vi "Untitled 6.vi"() -> ()   [LabVIEW 2017]
uses:
  <vilib>/myRIO/Instrument Drivers/Onboard IO/PWM/typedefs/PWM Reference.ctl
  <vilib>/myRIO/Common/Instrument Driver Framework/Utilities/typedefs/myRIO Generic Hardware Reference.ctl
  <vilib>/myRIO/Common/Instrument Driver Framework/Utilities/typedefs/Hardware Version Enum.ctl
  <vilib>/myRIO/Common/Instrument Driver Framework/Utilities/typedefs/myRIO v1.0 Reference.ctl
  <vilib>/myRIO/Common/Instrument Driver Framework/Utilities/typedefs/Generic FPGA Reference.ctl
  <vilib>/myRIO/Common/Instrument Driver Framework/myRIO v1.0/PWM/typedefs/PWM Channels Enum.ctl
  <vilib>/myRIO/Instrument Drivers/Onboard IO/PWM/typedefs/PWM Configuration.ctl
  <vilib>/userdefined/High Color/nirio_resource_hc.ctl
  <vilib>/myRIO/Instrument Drivers/Onboard IO/DIO/typedefs/DIO Reference.ctl
  <vilib>/myRIO/Common/Instrument Driver Framework/myRIO v1.0/DIO/typedefs/DIO Channels List.ctl
  <vilib>/myRIO/Common/Instrument Driver Framework/myRIO v1.0/DIO/typedefs/DIO Channels Enum.ctl
  <vilib>/myRIO/Common/Instrument Driver Framework/Utilities/vis/Is FPGA Ref Available.vi
  <vilib>/myRIO/Common/Instrument Driver Framework/myRIO v1.0/PWM/vis/myRIO v1.1 Open PWM.vi
  <vilib>/myRIO/Instrument Drivers/Onboard IO/PWM/vis/Set Duty Cycle and Frequency.vi
  <vilib>/myRIO/Common/Instrument Driver Framework/myRIO v1.0/DIO/vis/myRIO v1.1 Open DIO.vi
  <vilib>/myRIO/Common/Instrument Driver Framework/Utilities/vis/Validate Channels.vi
  <vilib>/myRIO/Common/Instrument Driver Framework/myRIO v1.0/PWM/vis/myRIO v1.0 Reserve PWM.vi
  <vilib>/myRIO/Common/Instrument Driver Framework/myRIO v1.0/DIO/vis/myRIO v1.0 Reserve DIO.vi
  <vilib>/myRIO/Common/Instrument Driver Framework/myRIO v1.0/DIO/vis/myRIO v1.0 Close DIO.vi
  <vilib>/myRIO/Common/Instrument Driver Framework/myRIO v1.0/UART/vis/myRIO v1.0 Close UART.vi
  <vilib>/myRIO/Common/Instrument Driver Framework/myRIO v1.0/PWM/vis/myRIO v1.0 Build MUX Configuration PWM.vi
  <vilib>/myRIO/Common/Instrument Driver Framework/myRIO v1.0/Resource Manager/vis/myRIO v1.0 Reserve Channel List.vi
  <vilib>/myRIO/Common/Instrument Driver Framework/myRIO v1.0/DIO/vis/myRIO v1.0 Build MUX Configuration DIO.vi
  <vilib>/myRIO/Common/Instrument Driver Framework/myRIO v1.0/DIO/vis/myRIO v1.0 Unreserve DIO.vi
  <vilib>/myRIO/Common/Instrument Driver Framework/myRIO v1.0/Resource Manager/vis/myRIO v1.0 Create Configuration List.vi
  <vilib>/myRIO/Common/Instrument Driver Framework/myRIO v1.0/Resource Manager/vis/myRIO v1.0 Reserve Channel.vi
  <vilib>/myRIO/Common/Instrument Driver Framework/myRIO v1.0/Resource Manager/vis/myRIO v1.0 Unreserve Channel.vi
  <vilib>/myRIO/Common/Instrument Driver Framework/myRIO v1.0/Resource Manager/vis/myRIO v1.0 Unreserve Channel List.vi
  <vilib>/myRIO/Common/Instrument Driver Framework/myRIO v1.0/Resource Manager/vis/myRIO v1.0 Build Mutex Name.vi
  <vilib>/Utility/VariantDataType/GetNumericInfo.vi
  <vilib>/Utility/error.llb/Error Cluster From Error Code.vi
  <vilib>/myRIO/Common/Instrument Driver Framework/myRIO v1.0/myRIO v1.1 Open.vi
  <vilib>/myRIO/Common/Instrument Driver Framework/Utilities/vis/IO Manager.vi
  <vilib>/myRIO/Common/Instrument Driver Framework/Utilities/vis/Configuration Manager.vi
  <vilib>/myRIO/Common/Instrument Driver Framework/myRIO v1.0/Resource Manager/vis/myRIO v1.0 Configure IO.vi
  <vilib>/myRIO/Common/Instrument Driver Framework/myRIO v1.0/myRIO v1.0 Close.vi
  <vilib>/myRIO/Common/Instrument Driver Framework/myRIO v1.0/PWM/vis/myRIO v1.0 Write PWM.vi
  <vilib>/myRIO/Common/Instrument Driver Framework/myRIO v1.0/DIO/vis/myRIO v1.0 Write DIO.vi
  <vilib>/myRIO/Common/Instrument Driver Framework/myRIO v1.0/DIO/vis/myRIO v1.0 Read DIO.vi
  <vilib>/myRIO/Common/Instrument Driver Framework/myRIO v1.0/DIO/vis/myRIO v1.0 Shutdown DIO.vi
  <vilib>/myRIO/Common/Instrument Driver Framework/Utilities/vis/FPGA Ref Manager.vi
  <vilib>/myRIO/Common/Instrument Driver Framework/myRIO v1.0/myRIO v1.0 Reset FPGA.vi
  <vilib>/myRIO/Common/Instrument Driver Framework/myRIO v1.0/IRQ/vis/myRIO v1.0 IRQ Info FGV.vi
  <vilib>/myRIO/Common/Instrument Driver Framework/myRIO v1.0/IRQ/vis/myRIO v1.0 Timer IRQ Info FGV.vi
  <vilib>/myRIO/Common/Instrument Driver Framework/myRIO v1.0/IRQ/vis/myRIO v1.0 ISR Agent.vi
  <vilib>/myRIO/Express VI/Onboard IO/PWM/PWM Express VI.xnode
  <vilib>/myRIO/Instrument Drivers/Onboard IO/PWM/vis/myRIO PWM Open.xnode
  <vilib>/myRIO/Express VI/Onboard IO/DO/DO Express VI.xnode
  <vilib>/myRIO/Instrument Drivers/Onboard IO/DIO/vis/myRIO DIO Open.xnode
  <vilib>/myRIO/Express VI/Onboard Devices/LED/LED Express VI.xnode
  <vilib>/myRIO/Instrument Drivers/Utilities/Utilities.lvlib
  <vilib>/myRIO/Instrument Drivers/Onboard IO/DIO/DIO.lvlib
  <vilib>/myRIO/Instrument Drivers/Onboard IO/PWM/PWM.lvlib
panel:
  in  "Angle":dbl
  in  "Numeric":dbl
  in  "error in (no error)":errorcluster
  in  "myRIO DIO Channel":tag="C/DIO1"
  in  "Temperature (deg C)":dbl=25.0
  out "Distance (cm)":dbl
  in  "stop":bool
  in  "fwd":bool
  out "error out":errorcluster
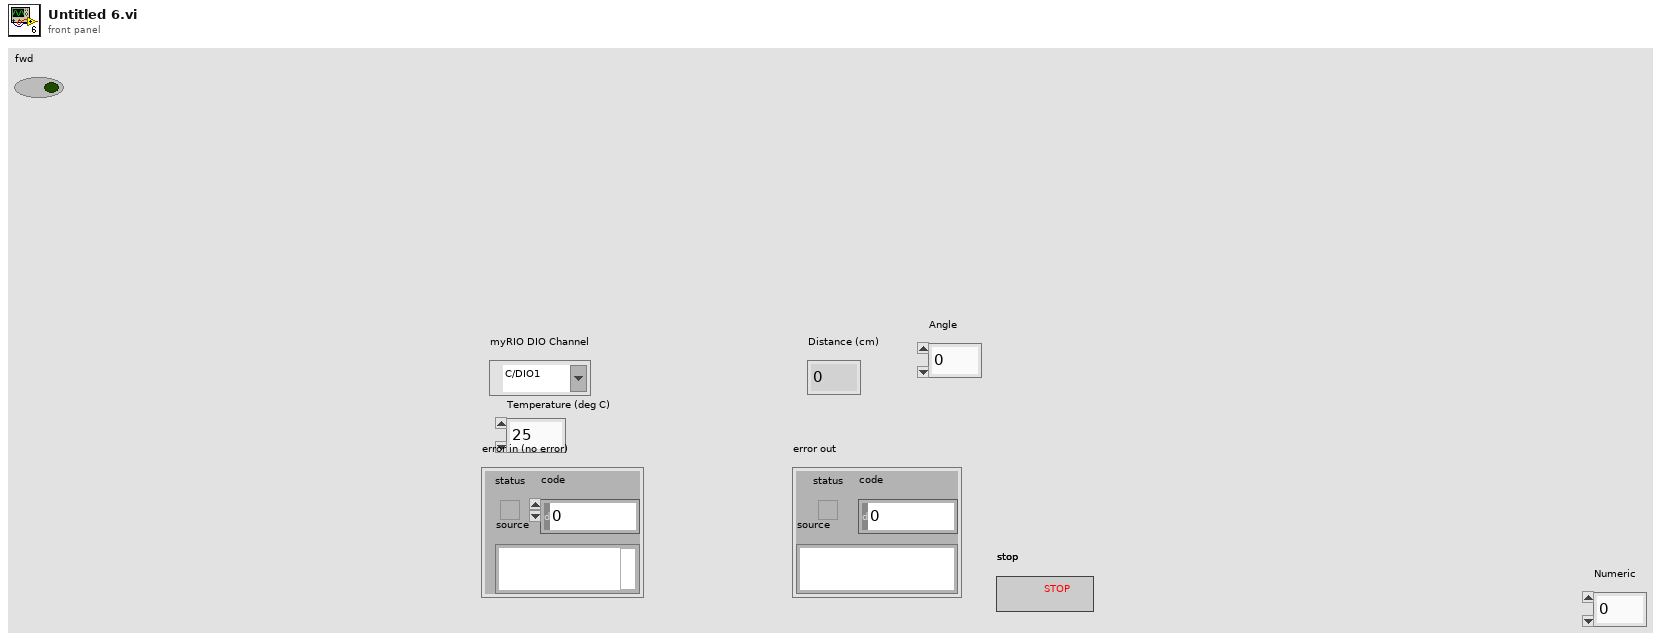
[diagram p1: front panel]
types:
  T1 = enum16{"Initialize", "Trigger pulse", "Wait for rising edge", "Wait for falling edge", "Calculate distance", "Stop"}
  T2 = typedef "DIO.lvlib/DIO Reference.ctl" = cluster{"myRIO Reference":T3, "DIO Channels List":T7}
  T3 = typedef "myRIO Generic Hardware Reference.ctl" = cluster{"myRIO Model":T4, "myRIO Hardware Reference":T5}
  T4 = typedef "Hardware Version Enum.ctl" = enum16{"Unknown", "myRIO-1900", "myRIO-1950", "roboRIO", "NI ELVIS RIO CM"}
  T5 = typedef "myRIO v1.0 Reference.ctl" = cluster{"Generic FPGA Reference":T6, "Allow multiple opens":bool}
  T6 = typedef "Generic FPGA Reference.ctl" = refnum<k20>
  T7 = typedef "DIO Channels List.ctl" = T8[]
  T8 = typedef "DIO Channels Enum.ctl" = enum16{"Not Connected", "C/DIO0", "C/DIO1", "C/DIO2", "C/DIO3", "C/DIO4", "C/DIO5", "C/DIO6", "C/DIO7", "A/DIO0", "A/DIO1", "A/DIO2", "A/DIO3", "A/DIO4", "A/DIO5", "A/DIO6", "A/DIO7", "A/DIO8", "A/DIO9", "A/DIO10", "A/DIO11", "A/DIO12", "A/DIO13", "A/DIO14", "A/DIO15", "B/DIO0", "B/DIO1", "B/DIO2", "B/DIO3", "B/DIO4", "B/DIO5", "B/DIO6", "B/DIO7", "B/DIO8", "B/DIO9", "B/DIO10", "B/DIO11", "B/DIO12", "B/DIO13", "B/DIO14", "B/DIO15", "LED0", "LED1", "LED2", "LED3", "Button0", "DIO/DIO0", "DIO/DIO1", "DIO/DIO2", "DIO/DIO3", "DIO/DIO4", "DIO/DIO5", "DIO/DIO6", "DIO/DIO7", "DIO/DIO8", "DIO/DIO9", "SPI/CS0", "SPI/CS1", "SPI/CS2", "SPI/CS3", "LED RADIO (Green)", "LED RADIO (Red)", "LED COMM (Green)", "LED COMM (Red)", "LED MODE (Green)", "LED MODE (Red)"}
  T9 = typedef "nirio_resource_hc.ctl" = tag
  T10 = typedef "PWM.lvlib/PWM Reference.ctl" = cluster{"myRIO Reference":T3, "PWM Channels Enum":T11, "PWM Configuration":T12}
  T11 = typedef "PWM Channels Enum.ctl" = enum16{"Not Connected", "C/PWM0", "C/PWM1", "A/PWM0", "A/PWM1", "A/PWM2", "B/PWM0", "B/PWM1", "B/PWM2", "PWM/PWM0", "PWM/PWM1", "PWM/PWM2", "PWM/PWM3", "PWM/PWM4", "PWM/PWM5", "PWM/PWM6", "PWM/PWM7", "PWM/PWM8", "PWM/PWM9"}
  T12 = typedef "PWM.lvlib/PWM Configuration.ctl" = cluster{"Frequency":dbl, "Duty Cycle":dbl}
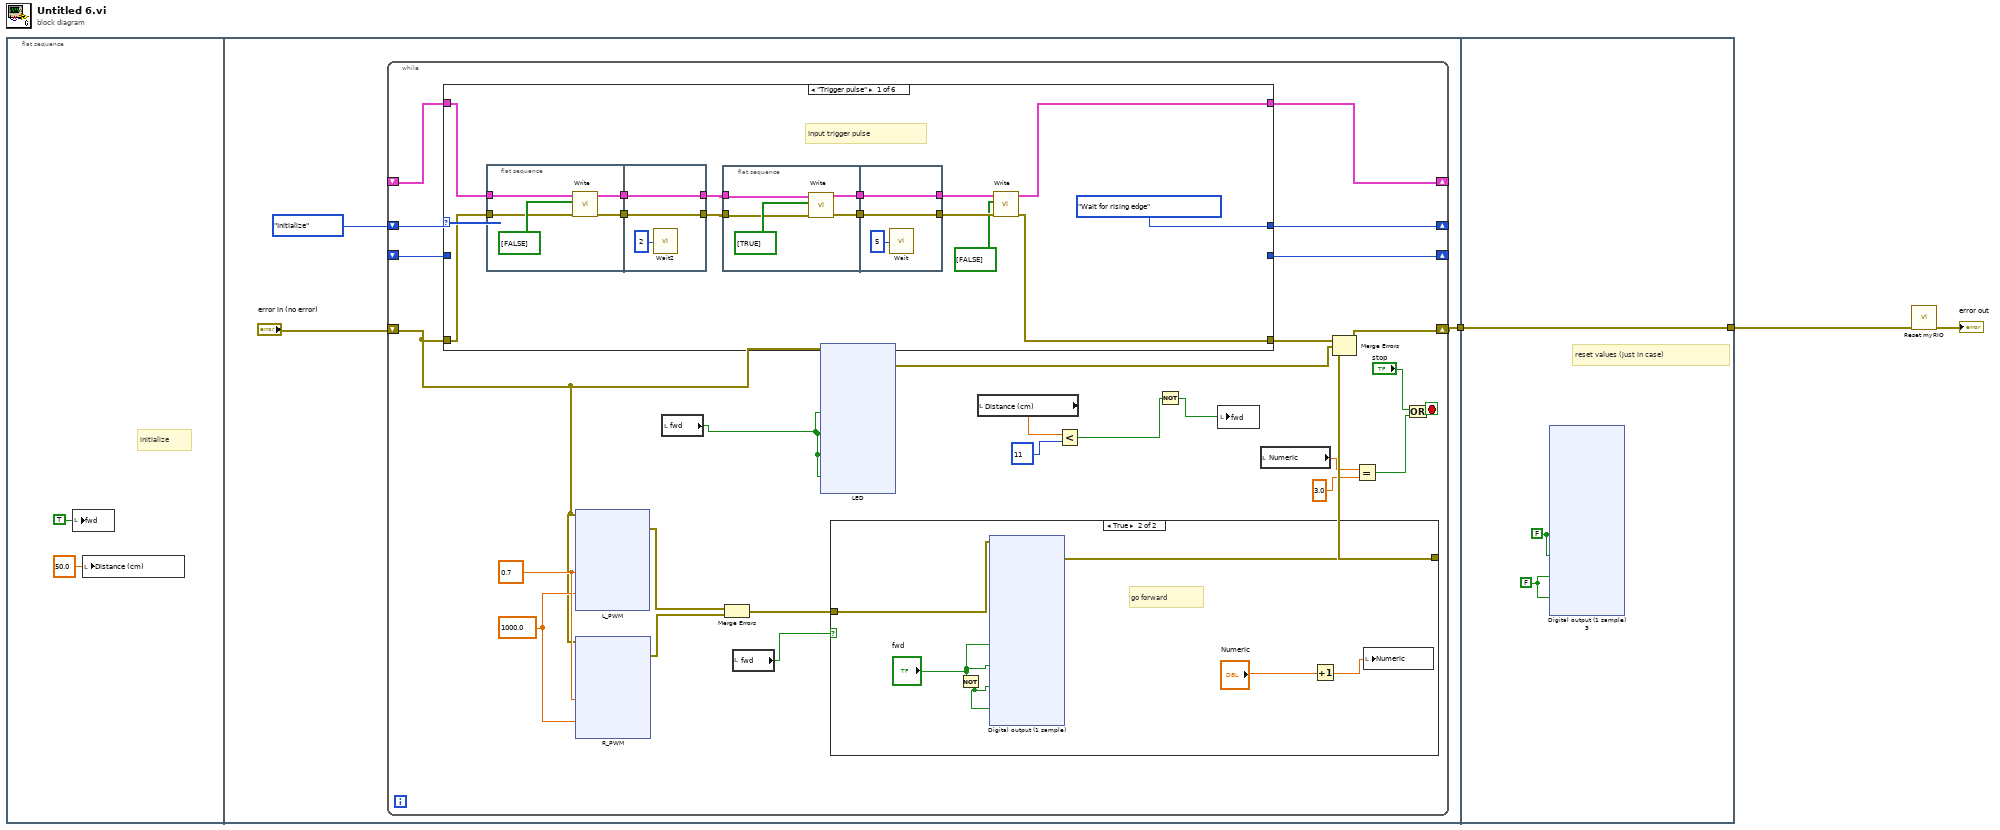
[diagram p0: block diagram]
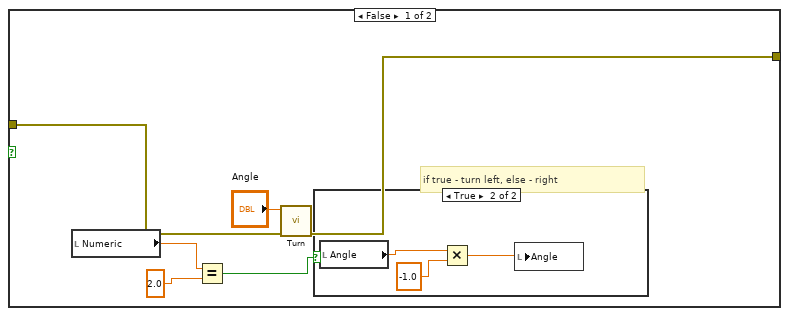
[diagram p2: hidden frame]
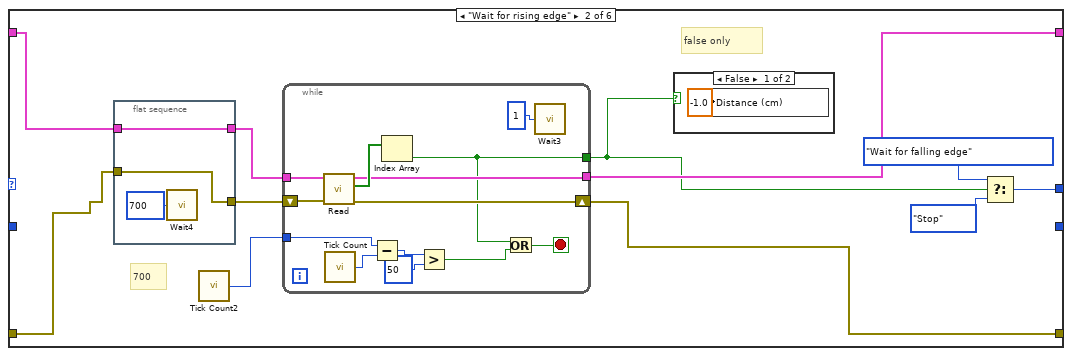
[diagram p4: hidden frame]
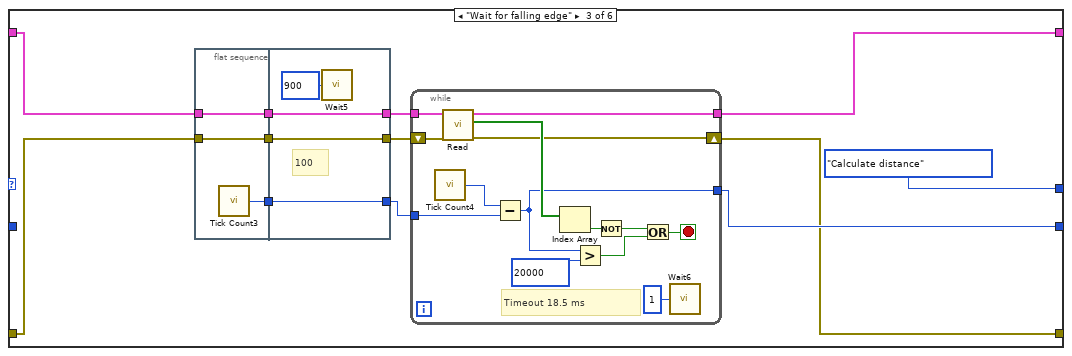
[diagram p6: hidden frame]
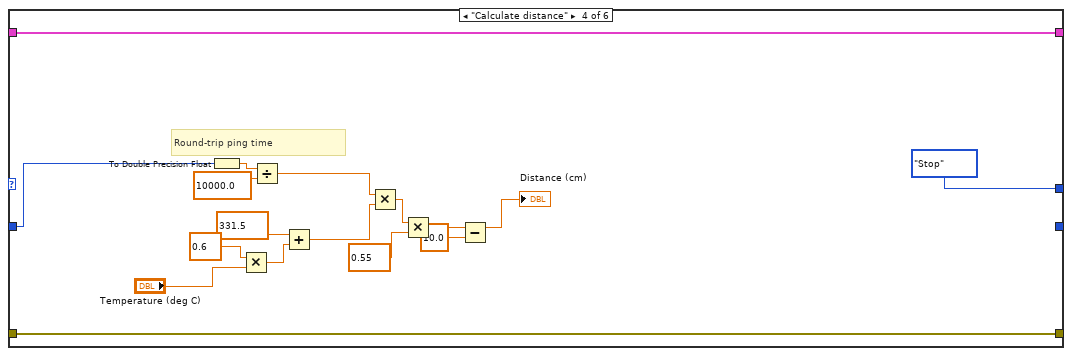
[diagram p7: hidden frame]
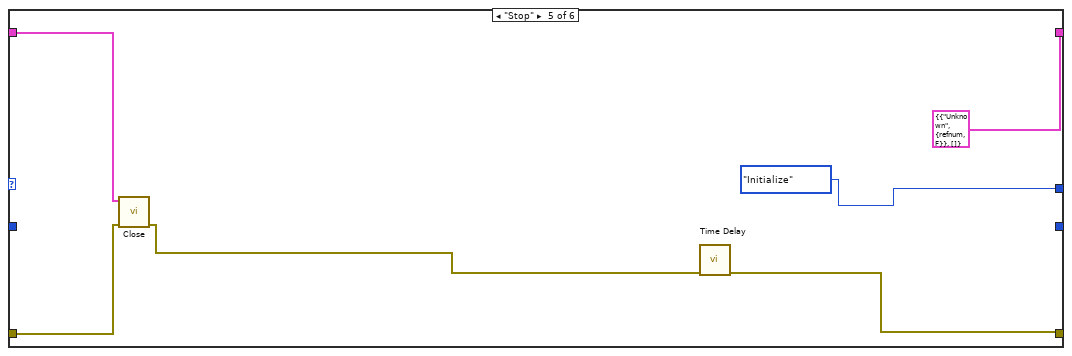
[diagram p8: hidden frame]
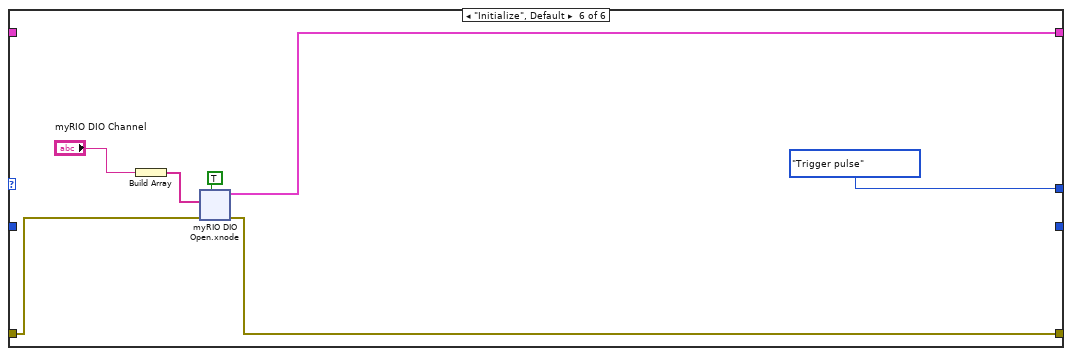
[diagram p9: hidden frame]
diagram:
  n1 = flat-sequence {
    tunnel: [w6] -> w1
    tunnel: [w336] -> w3
    tunnel: w1 -> [w336]
    frame #0 {
      # "initialize"
      n2 = local write "fwd"(TRUE ("fwd")) -> ()
      n3 = local write "Distance (cm)"(50.0 ("Distance (cm)")) -> ()
    }
    frame #1 {
      n4 = while {
        shift-right: [w30] -> _
        shift-left: T1."Initialize" -> [w35]
        shift-right: [w27] -> w6
        shift-left: "error in (no error)" -> [w19]
        shift-right: [w34] -> _
        shift-left: _ -> [w33]
        shift-right: [w29] -> _
        shift-left: _ -> [w31]
        stop <- w18 stop-if-true
        w22 = 1000.0 ("Frequency [Hz]")
        w23 = 0.7 ("Duty Cycle")
        n5 = case shown="\"Trigger pulse\"" w35 {
          tunnel: [T1."Wait for rising edge" w228 T1."Calculate distance" ("y") T1."Stop" ("y") T1."Initialize" ("y") T1."Trigger pulse"] -> w30
          tunnel: w19 -> [w201 w233 w259 w292 w310 w315]
          tunnel: [w199 w237 w258 w304 T2 {"myRIO Reference"={"myRIO Model"=enum."Unknown", "myRIO Hardware Reference"={"Generic FPGA Reference"=refnum, "Allow multiple opens"=FALSE}}, "DIO Channels List"=[]} ("DIO Ref Out") w314] -> w34
          tunnel: w33 -> [w200 w232 w260 w304 w309 _]
          tunnel: [w198 w236 w255 w292 w305 w313] -> w32
          tunnel: [_ _ w257 _ _ _] -> w29
          tunnel: w31 -> [_ _ _ w291 _ _]
          frame "Trigger pulse" {
            # "Input trigger pulse"
            n6 = flat-sequence {
              tunnel: [w214] -> w208
              tunnel: [w213] -> w207
              tunnel: w201 -> [w212]
              tunnel: w200 -> [w211]
              tunnel: [w217] -> w205
              tunnel: [w216] -> w206
              tunnel: w208 -> [w217]
              tunnel: w207 -> [w216]
              frame #0 {
                n7 = call <vilib>:"Write.vi"("error in (no error)"=w212, "Values"=bool[] [FALSE], "DIO Ref In"=w211) -> ("error out"=w213:errorcluster, "DIO Ref Out"=w214:T2)  [unwired: 6 in]
              }
              frame #1 {
                n8 = call "Wait2"("Count(uSec)"=u32 2) -> ()  [unwired: 1 out]
              }
            }
            n9 = flat-sequence {
              tunnel: [w222] -> w210
              tunnel: [w221] -> w209
              tunnel: w206 -> [w220]
              tunnel: w205 -> [w219]
              tunnel: [w225] -> w202
              tunnel: [w224] -> w204
              tunnel: w210 -> [w225]
              tunnel: w209 -> [w224]
              frame #0 {
                n10 = call <vilib>:"Write.vi"("error in (no error)"=w220, "Values"=bool[] [TRUE], "DIO Ref In"=w219) -> ("error out"=w221:errorcluster, "DIO Ref Out"=w222:T2)  [unwired: 6 in]
              }
              frame #1 {
                n11 = call "Wait"("Count(uSec)"=u32 5) -> ()  [unwired: 1 out]
              }
            }
            n12 = call <vilib>:"Write.vi"("error in (no error)"=w204, "Values"=bool[] [FALSE], "DIO Ref In"=w202) -> ("error out"=w198:errorcluster, "DIO Ref Out"=w199:T2)  [unwired: 6 in]
          }
          frame "Wait for rising edge" {
            # "700"
            # "false only"
            n13 = flat-sequence {
              tunnel: [w240] -> w234
              tunnel: w233 -> [w240]
              tunnel: w232 -> [w239]
              tunnel: [w239] -> w231
              frame #0 {
                n14 = call "Wait4"("Count(uSec)"=u32 700) -> ()  [unwired: 1 out]
              }
            }
            n15 = call "Tick Count2"() -> ("Tick Count(uSec)"=w235:u32)
            n16 = while {
              tunnel: [w252] -> w237
              shift-right: [w250] -> w236
              shift-left: w234 -> [w251]
              tunnel: w235 -> [w247]
              tunnel: w231 -> [w249]
              tunnel: [w242] -> w227
              stop <- w244 stop-if-true
              n17 = call <vilib>:"Read.vi"("error in (no error)"=w251, "DIO Ref In"=w249) -> ("error out"=w250:errorcluster, "Values"=w253:bool[], "DIO Ref Out"=w252:T2)  [unwired: 7 in]
              n18 = call "Tick Count"() -> ("Tick Count(uSec)"=w248:u32)
              n19 = Subtract(x=w247, y=w248) -> (x-y=w246:u32)
              n20 = Index Array(array=w253) -> (element=w242:bool)  [unwired: 1 in]
              n21 = Greater?(x=w246, y=u32 50) -> (0:w243:bool)
              n22 = Or(x=w242, y=w243) -> (x .or. y?=w244:bool)
              n23 = call "Wait3"("Count(uSec)"=u32 1) -> ()  [unwired: 1 out]
            }
            n24 = case shown="False" w227 {
              frame False {
                n25 = local write "Distance (cm)"(-1.0 ("Distance (m)")) -> ()
              }
              frame True {
              }
            }
            n26 = Select(t=T1."Wait for falling edge", s=w227, f=T1."Stop" ("y")) -> (s? t:f=w228:T1)
          }
          frame "Wait for falling edge" {
            n27 = flat-sequence {
              tunnel: w260 -> [w283]
              tunnel: [w283] -> w266
              tunnel: [w282] -> w265
              tunnel: [w281] -> w264
              tunnel: w259 -> [w281]
              tunnel: [w286] -> w262
              tunnel: [w287] -> w263
              tunnel: w266 -> [w287]
              tunnel: w265 -> [w286]
              tunnel: w264 -> [w284]
              tunnel: [w284] -> w261
              frame #0 {
                n28 = call "Tick Count3"() -> ("Tick Count(uSec)"=w282:u32)
              }
              frame #1 {
                # "100"
                n29 = call "Wait5"("Count(uSec)"=u32 900) -> ()  [unwired: 1 out]
              }
            }
            n30 = while {
              tunnel: w263 -> [w279]
              tunnel: w262 -> [w276]
              shift-right: [w270] -> w255
              shift-left: w261 -> [w271]
              tunnel: [w268] -> w258
              tunnel: [w267] -> w257
              stop <- w275 stop-if-true
              # "Timeout 18.5 ms"
              n31 = call "Tick Count4"() -> ("Tick Count(uSec)"=w269:u32)
              n32 = call <vilib>:"Read.vi"("error in (no error)"=w271, "DIO Ref In"=w279) -> ("error out"=w270:errorcluster, "Values"=w278:bool[], "DIO Ref Out"=w268:T2)  [unwired: 7 in]
              n33 = Subtract(x=w269, y=w276) -> (x-y=w267:u32)
              n34 = Index Array(array=w278) -> (element=w277:bool)  [unwired: 1 in]
              n35 = Greater?(x=w267, y=u32 20000) -> (0:w273:bool)
              n36 = Not(x=w277) -> (.not. x?=w274:bool)
              n37 = Or(x=w274, y=w273) -> (x .or. y?=w275:bool)
              n38 = call "Wait6"("Count(uSec)"=u32 1) -> ()  [unwired: 1 out]
            }
          }
          frame "Calculate distance" {
            # "Round-trip ping time"
            n39 = To Double Precision Float(number=w291) -> (double precision float=w299:dbl)
            n40 = Multiply(x=0.6, y="Temperature (deg C)") -> (x*y=w297:dbl)
            n41 = Divide(x=w299, y=10000.0) -> (x/y=w301:dbl)
            n42 = Add(x=331.5, y=w297) -> (x+y=w302:dbl)
            n43 = Multiply(x=w301, y=w302) -> (x*y=w294:dbl)
            n44 = Multiply(x=w294, y=0.55) -> (x*y=w290:dbl)
            n45 = Subtract(x=w290, y=10.0) -> (x-y=→"Distance (cm)":dbl)
          }
          frame "Stop" {
            n46 = call <vilib>:"Close.vi"("error in (no error)"=w310, "DIO Ref In"=w309) -> ("error out"=w306:errorcluster)  [unwired: 9 in]
            n47 = call "Time Delay"("error in (no error)"=w306) -> ("error out"=w305:errorcluster)  [unwired: 10 in]
          }
          frame "Initialize", Default {
            n48 = Build Array("myRIO DIO Channel") -> (w317:tag[])
            n49 = xnode "myRIO DIO Open.xnode"("error in (no error)"=w315, "Allow multiple opens?"=TRUE, "Channel Names"=w317) -> ("error out"=w313:errorcluster, "DIO Ref Out"=w314:T2)
          }
        }
        n50 = xnode "L_PWM"("Duty Cycle"=w23, "Frequency [Hz]"=w22, "error in (no error)"=w19) -> ("error out"=w24:errorcluster)
        n51 = xnode "R_PWM"("Duty Cycle"=w23, "Frequency [Hz]"=w22, "error in (no error)"=w19) -> ("error out"=w25:errorcluster)
        n52 = local read "fwd"() -> (w17:bool)
        n53 = Merge Errors(w24, w25) -> (w21:errorcluster)
        n54 = local read "fwd"() -> (w12:bool)
        n55 = xnode "LED"("LED0"=w17, "LED1"=w17, "LED2"=w17, "LED3"=w17, "error in (no error)"=w19) -> ("error out"=w26:errorcluster)
        n56 = case shown="True" w12 {
          tunnel: w21 -> [w41 w50]
          tunnel: [w40 w49] -> w20
          frame False {
            # "if true - turn left, else - right"
            n57 = local read "Numeric"() -> (w39:dbl)
            n58 = Equal?(x=w39, y=2.0) -> (x = y?=w36:bool)
            n59 = call "Turn.vi"("error in (no error)"=w41, "Angle"="Angle") -> ("error out"=w40:errorcluster)  [unwired: 9 in]
            n60 = case shown="True" w36 {
              frame False {
              }
              frame True {
                n61 = local read "Angle"() -> (w44:dbl)
                n62 = Multiply(x=w44, y=-1.0) -> (x*y=w42:dbl)
                n63 = local write "Angle"(w42) -> ()
              }
            }
          }
          frame True {
            # "go forward"
            n64 = Not(x="fwd") -> (.not. x?=w47:bool)
            n65 = xnode "Digital output (1 sample)"("Left+ (A/DIO5 (Pin 21))"="fwd", "Right+ (A/DIO7 (Pin 25))"="fwd", "Left- (A/DIO6 (Pin 23))"=w47, "Right- (A/DIO13 (Pin 26))"=w47, "error in (no error)"=w50) -> ("error out"=w49:errorcluster)
            n66 = Increment(x="Numeric") -> (x+1=w46:dbl)
            n67 = local write "Numeric"(w46) -> ()
          }
        }
        n68 = local read "Distance (cm)"() -> (w15:dbl)
        n69 = Less?(x=w15, y=11) -> (x < y?=w16:bool)
        n70 = Not(x=w16) -> (.not. x?=w14:bool)
        n71 = local write "fwd"(w14) -> ()
        n72 = local read "Numeric"() -> (w11:dbl)
        n73 = Merge Errors(w32, w26, w20) -> (w27:errorcluster)
        n74 = Equal?(x=w11, y=3.0) -> (x = y?=w9:bool)
        n75 = Or(x="stop", y=w9) -> (x .or. y?=w18:bool)
      }
    }
    frame #2 {
      w334 = FALSE ("Left+ (A/DIO5 (Pin 21))")
      w335 = FALSE ("Left+ (A/DIO5 (Pin 21))")
      # "reset values (just in case)"
      n76 = xnode "Digital output (1 sample) 3"("Left+ (A/DIO5 (Pin 21))"=w335, "Right+ (A/DIO7 (Pin 25))"=w335, "Left- (A/DIO6 (Pin 23))"=w334, "Right- (A/DIO13 (Pin 26))"=w334) -> ()  [unwired: 1 in, 1 out]
    }
  }
  n77 = call <vilib>:"Reset myRIO.vi"("error in (no error)"=w3) -> ("error out"=→"error out":errorcluster)  [unwired: 10 in]
